vi "Lock-in update.vi"(8 "error in (no error)":errorcluster, 11 "Lock-in Handle":T2 {"Handle" format="0x%08x"; "Conn" format="0x%08x"}) -> (0 "error out":errorcluster, 1 "Lock-in info":T1, 3 "Handle Out":T2 {"Handle" format="0x%08x"; "Conn" format="0x%08x"})   [LabVIEW 2024, in "Lock-in module.lvlib"]
uses:
  Lock-in module.lvlib
  <instrlib>/Zurich Instruments LabOne/Public/ziTypeHandle.ctl
  ctl/ACQ info.ctl
  <instrlib>/Zurich Instruments LabOne/Public/Configure/ziGetValueDouble.vi
  <instrlib>/Zurich Instruments LabOne/Zurich Instruments LabOne.lvlib
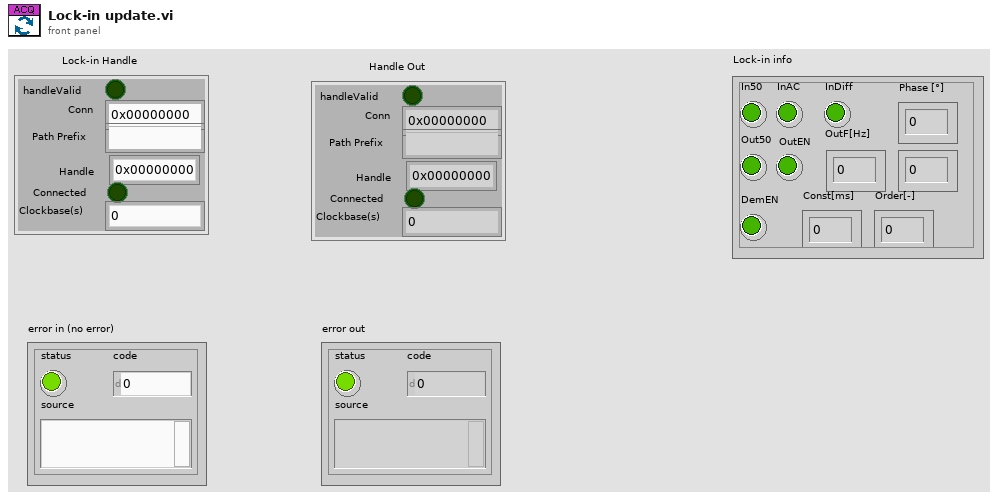
[diagram p1: front panel]
types:
  T1 = typedef "Lock-in module.lvlib/ACQ info.ctl" = cluster{"In50":bool, "InAC":bool, "InDiff":bool, "Out50":bool, "OutEN":bool, "OutF[Hz]":dbl, "OutA[V]":dbl, "DemEN":bool, "Const[ms]":dbl, "Order[-]":i32, "Phase [°]":dbl}
  T2 = typedef "Zurich Instruments LabOne.lvlib/ziTypeHandle.ctl" = cluster{"handleValid":bool, "Conn":u64, "Path Prefix":string, "Handle":u64, "Connected":bool, "Clockbase(s)":dbl}
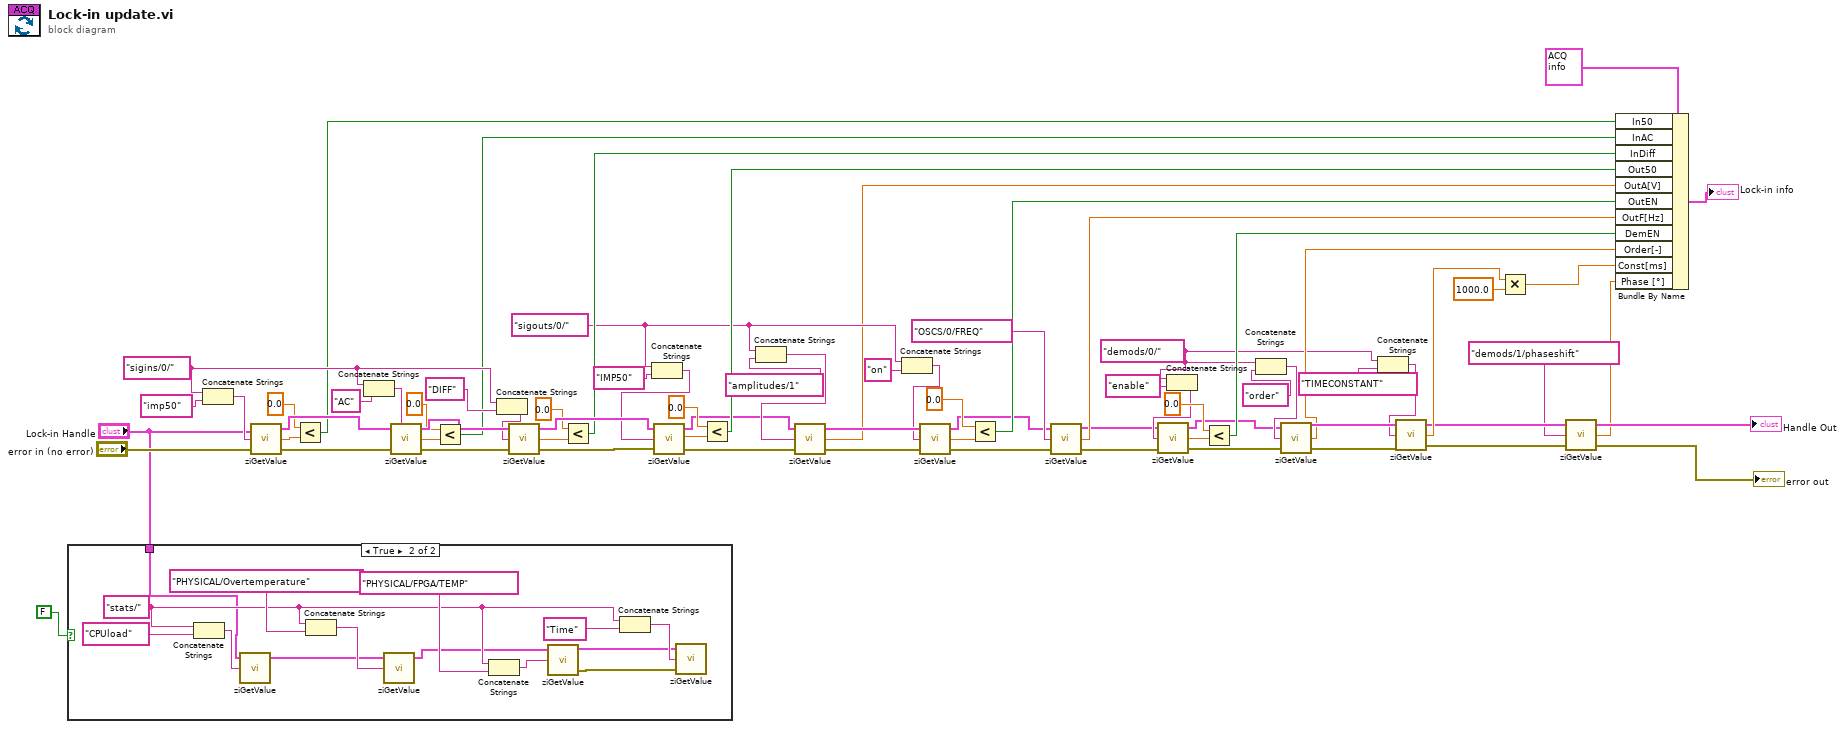
[diagram p0: block diagram]
diagram:
  w10 = "demods/0/"
  w38 = "sigouts/0/" ("string")
  w70 = "sigins/0/"
  n1 = case shown="True" FALSE {
    tunnel: "Lock-in Handle" -> [_ w76]
    frame False {
    }
    frame True {
      w83 = "stats/" ("Path")
      n2 = Concatenate Strings(w83, "CPUload") -> (w86:string)
      n3 = call-poly <instrlib>:"ziGetValue.vi"("Path"=w86, "Handle in"=w76) -> ("Handle out"=w78:T2)  [unwired: 1 in, 2 out]
      n4 = Concatenate Strings(w83, "PHYSICAL/Overtemperature") -> (w88:string)
      n5 = call-poly <instrlib>:"ziGetValue.vi"("Path"=w88, "Handle in"=w78) -> ("Handle out"=w79:T2)  [unwired: 1 in, 2 out]
      n6 = Concatenate Strings(w83, "PHYSICAL/FPGA/TEMP") -> (w84:string)
      n7 = call-poly <instrlib>:"ziGetValue.vi"("Path"=w84, "Handle in"=w79) -> ("error out"=w81:errorcluster, "Handle out"=w77:T2)  [unwired: 1 in, 1 out]
      n8 = Concatenate Strings(w83, "Time") -> (w80:string)
      n9 = call-poly <instrlib>:"ziGetValue.vi"("error in"=w81, "Path"=w80, "Handle in"=w77) -> ()  [unwired: 3 out]
    }
  }
  n10 = Concatenate Strings(w70, "imp50" ("Path")) -> (w67:string)
  n11 = call-poly <instrlib>:"ziGetValue.vi"("error in"="error in (no error)", "Path"=w67, "Handle in"="Lock-in Handle") -> ("error out"=w58:errorcluster, "Value"=w49:dbl, "Handle out"=w74:T2)
  n12 = Less?(x=0.0 ("y"), y=w49) -> (x < y?=w48:bool)
  n13 = Concatenate Strings(w70, "AC" ("Path")) -> (w66:string)
  n14 = call-poly <instrlib>:"ziGetValue.vi"("error in"=w58, "Path"=w66, "Handle in"=w74) -> ("error out"=w59:errorcluster, "Value"=w46:dbl, "Handle out"=w73:T2)
  n15 = Less?(x=0.0 ("y"), y=w46) -> (x < y?=w43:bool)
  n16 = Concatenate Strings(w70, "DIFF" ("Path")) -> (w65:string)
  n17 = call-poly <instrlib>:"ziGetValue.vi"("error in"=w59, "Path"=w65, "Handle in"=w73) -> ("error out"=w60:errorcluster, "Value"=w44:dbl, "Handle out"=w72:T2)
  n18 = Less?(x=0.0 ("y"), y=w44) -> (x < y?=w42:bool)
  n19 = Concatenate Strings(w38, "IMP50" ("Path")) -> (w61:string)
  n20 = call-poly <instrlib>:"ziGetValue.vi"("error in"=w60, "Path"=w61, "Handle in"=w72) -> ("error out"=w32:errorcluster, "Value"=w40:dbl, "Handle out"=w33:T2)
  n21 = Less?(x=0.0 ("y"), y=w40) -> (x < y?=w39:bool)
  n22 = Concatenate Strings(w38, "amplitudes/1") -> (w54:string)
  n23 = call-poly <instrlib>:"ziGetValue.vi"("error in"=w32, "Path"=w54, "Handle in"=w33) -> ("error out"=w57:errorcluster, "Value"=w34:dbl, "Handle out"=w56:T2)
  n24 = Concatenate Strings(w38, "on" ("Path")) -> (w53:string)
  n25 = call-poly <instrlib>:"ziGetValue.vi"("error in"=w57, "Path"=w53, "Handle in"=w56) -> ("error out"=w30:errorcluster, "Value"=w36:dbl, "Handle out"=w31:T2)
  n26 = Less?(x=0.0 ("y"), y=w36) -> (x < y?=w35:bool)
  n27 = call-poly <instrlib>:"ziGetValue.vi"("error in"=w30, "Path"="OSCS/0/FREQ", "Handle in"=w31) -> ("error out"=w23:errorcluster, "Value"=w29:dbl, "Handle out"=w24:T2)
  n28 = Concatenate Strings(w10, "enable" ("Path")) -> (w25:string)
  n29 = call-poly <instrlib>:"ziGetValue.vi"("error in"=w23, "Path"=w25, "Handle in"=w24) -> ("error out"=w15:errorcluster, "Value"=w27:dbl, "Handle out"=w18:T2)
  n30 = Less?(x=0.0 ("y"), y=w27) -> (x < y?=w22:bool)
  n31 = Concatenate Strings(w10, "order" ("string")) -> (w19:string)
  n32 = call-poly <instrlib>:"ziGetValue.vi"("error in"=w15, "Path"=w19, "Handle in"=w18) -> ("error out"=w14:errorcluster, "Value"=w11:dbl, "Handle out"=w16:T2)
  n33 = Concatenate Strings(w10, "TIMECONSTANT" ("string")) -> (w13:string)
  n34 = call-poly <instrlib>:"ziGetValue.vi"("error in"=w14, "Path"=w13, "Handle in"=w16) -> ("error out"=w3:errorcluster, "Value"=w9:dbl, "Handle out"=w6:T2)
  n35 = Multiply(x=w9, y=1000.0) -> (x*y=w7:dbl)
  n36 = call-poly <instrlib>:"ziGetValue.vi"("error in"=w3, "Path"="demods/1/phaseshift", "Handle in"=w6) -> ("error out"=→"error out":errorcluster, "Value"=w1:dbl, "Handle out"=→"Handle Out":T2)
  n37 = Bundle By Name(cluster=T1 {"In50"=FALSE, "InAC"=FALSE, "InDiff"=FALSE, "Out50"=FALSE, "OutEN"=FALSE, "OutF[Hz]"=0.0, "OutA[V]"=0.0, "DemEN"=FALSE, "Const[ms]"=0.0, "Order[-]"=0, "Phase [°]"=0.0} ("Cluster"), "In50"=w48, "InAC"=w43, "InDiff"=w42, "Out50"=w39, "OutA[V]"=w34, "OutEN"=w35, "OutF[Hz]"=w29, "DemEN"=w22, "Order[-]"=w11, "Const[ms]"=w7, "Phase [°]"=w1) -> (→"Lock-in info":T1)
